vi "In_S2F23.vi"(8 "error in (no error)":errorcluster, 11 "S2 Message Class in":refnum<class "S2 Message Class.lvclass">) -> (0 "error out":errorcluster, 1 "OK?":bool, 2 "S2F23":T1, 3 "S2 Message Class out":refnum<class "S2 Message Class.lvclass">)   [LabVIEW 2020, in "SECS Communication.lvlib" / "S2 Message Class.lvclass"]
uses:
  S2 Message Class.lvclass
  D:/Dropbox/SECS/SECS_GEM v1.0.6/Com/SECS Communication/SECS-II Class/SECS-II Class.lvclass
  S2F23.ctl
  SECS-II Class/SECS-II Class.lvclass/SECS-II Class.ctl
  SECS-II Class/Variant To Data_U4.vi
  SECS-II Class/Variant To Data_ASCII.vi
  SECS-II Class/SECS-II Class.lvclass
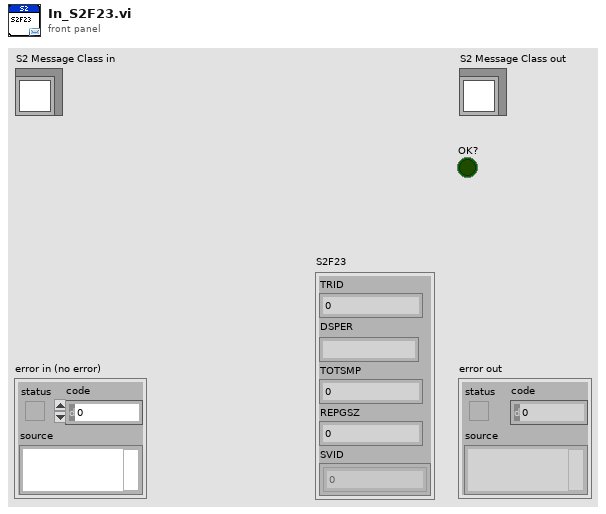
[diagram p1: front panel]
types:
  T1 = typedef "SECS Communication.lvlib/S2 Message Class.lvclass/S2F23.ctl" = cluster{"TRID":u32, "DSPER":string, "TOTSMP":u32, "REPGSZ":u32, "SVID":u32[]}
  T2 = typedef "SECS Communication.lvlib/SECS-II Class.lvclass/Message Data.ctl" = cluster{"Index":i32, "Data Item Format":T3, "Format Code":T4, "Parent Index":i32, "Child Index":i32[], "Data":variant}
  T3 = typedef "SECS Communication.lvlib/SECS-II Class.lvclass/Data Item Format.ctl" = enum16{"Data Type", "Value"}
  T4 = typedef "SECS Communication.lvlib/SECS-II Class.lvclass/Format Code.ctl" = enum16{"L", "A", "B", "Boolean", "J", "I1", "I2", "I4", "I8", "U1", "U2", "U4", "U8", "F4", "F8", "Char"}
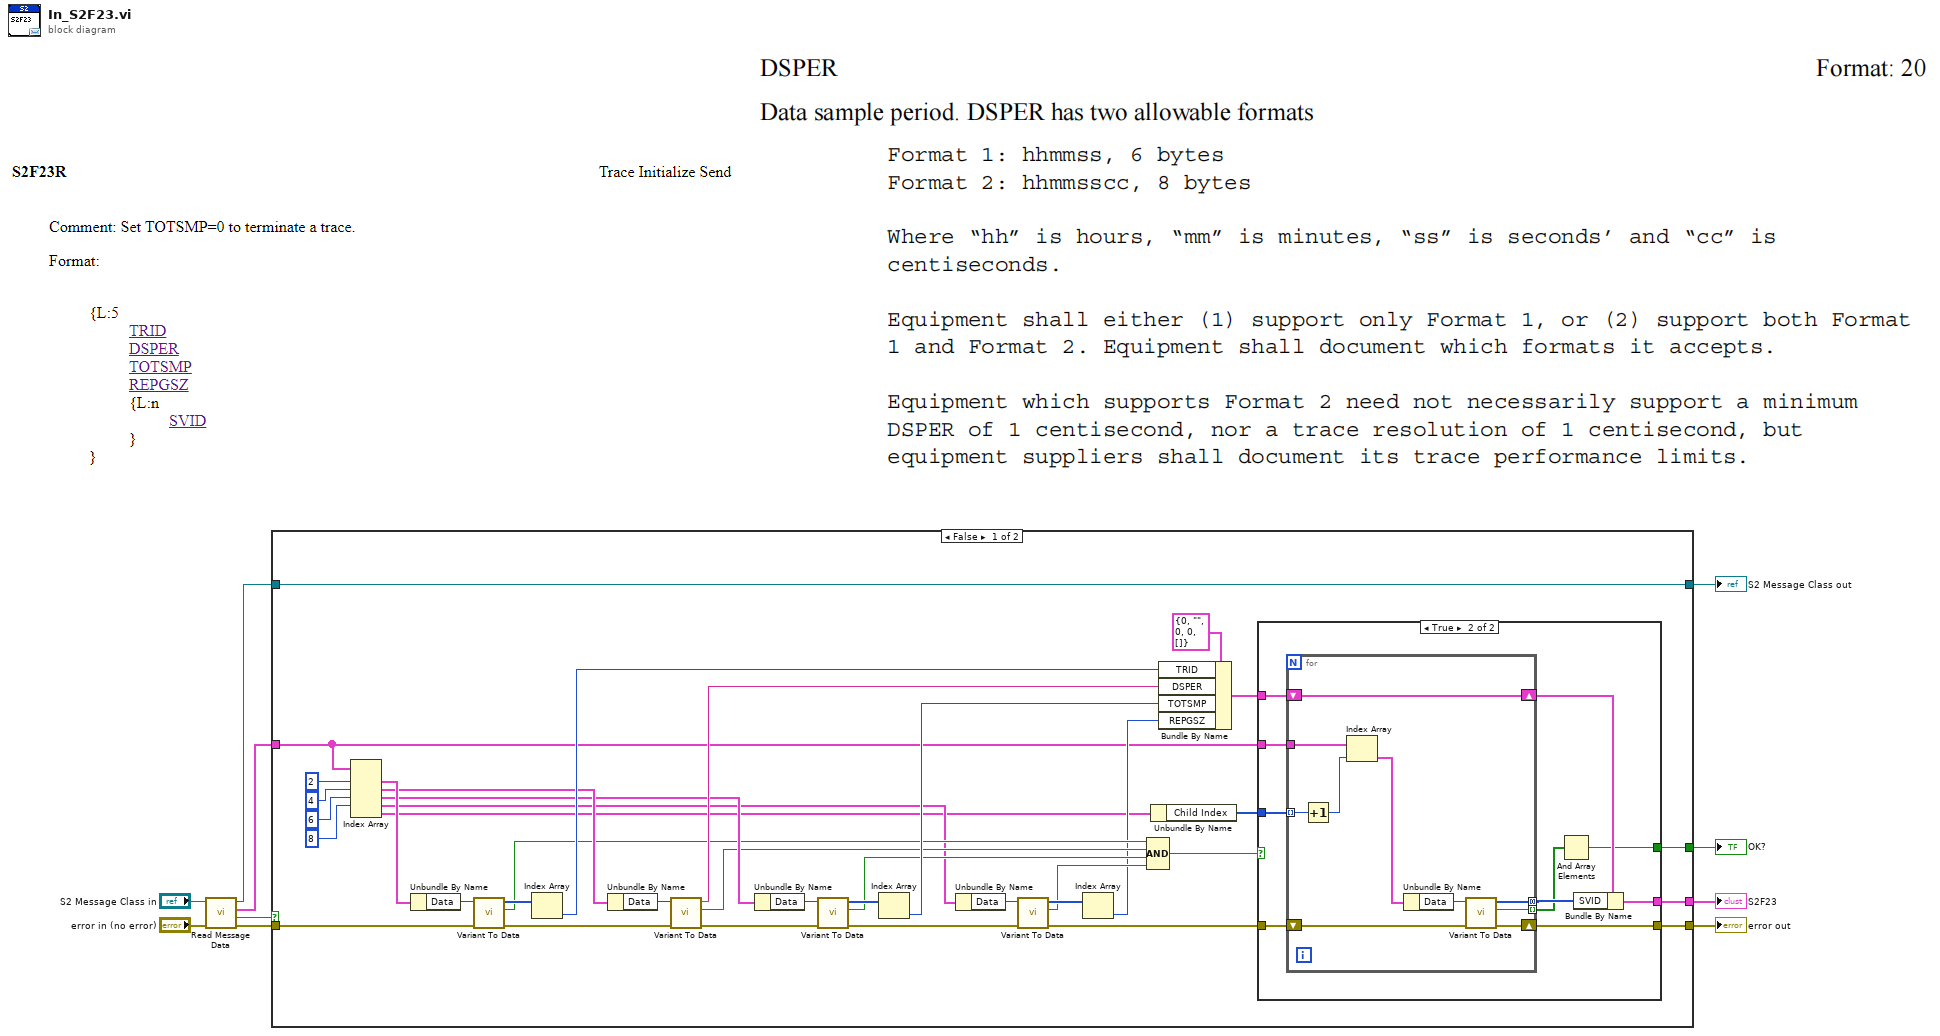
[diagram p0: block diagram]
diagram:
  n1 = call "Read Message Data.vi"("error in (no error)"="error in (no error)", "SECS-II Class in"="S2 Message Class in") -> ("error out"=w10:errorcluster, "Empty?"=w9:bool, "Message Data"=w8:T2[], "SECS-II Class out"=w7:refnum<class "S2 Message Class.lvclass">)  [unwired: 6 in]
  n2 = case shown="False" w9 {
    tunnel: w8 -> [w14 _]
    tunnel: w10 -> [w48 w70]
    tunnel: [w13 w70] -> w5
    tunnel: w7 -> [w47 w71]
    tunnel: [w47 w71] -> w1
    tunnel: [w12 _] -> w4
    tunnel: [w11 _] -> w6
    frame False {
      n3 = Index Array(array=w14, index #1=2 ("index"), index #2=4 ("index"), index #3=6 ("index"), index #4=8 ("index")) -> (element #1=w46:T2, element #2=w37:T2, element #3=w32:T2, element #4=w21:T2, element #5=w17:T2)  [unwired: 1 in]
      n4 = Unbundle By Name(w46) -> ("Data"=w45:variant)
      n5 = call-poly "Variant To Data.vi"("error in (no error)"=w48, "Variant"=w45) -> ("error out"=w38:errorcluster, "OK?"=w29:bool, "Data"=w42:u32[])  [unwired: 7 in]
      n6 = Index Array(array=w42) -> (element=w41:u32)  [unwired: 1 in]
      n7 = Unbundle By Name(w37) -> ("Data"=w39:variant)
      n8 = call-poly "Variant To Data.vi"("error in (no error)"=w38, "Variant"=w39) -> ("error out"=w34:errorcluster, "OK?"=w28:bool, "Data"=w36:string)  [unwired: 7 in]
      n9 = Unbundle By Name(w32) -> ("Data"=w35:variant)
      n10 = call-poly "Variant To Data.vi"("error in (no error)"=w34, "Variant"=w35) -> ("error out"=w23:errorcluster, "OK?"=w27:bool, "Data"=w30:u32[])  [unwired: 7 in]
      n11 = Index Array(array=w30) -> (element=w31:u32)  [unwired: 1 in]
      n12 = Unbundle By Name(w21) -> ("Data"=w24:variant)
      n13 = call-poly "Variant To Data.vi"("error in (no error)"=w23, "Variant"=w24) -> ("error out"=w19:errorcluster, "OK?"=w22:bool, "Data"=w25:u32[])  [unwired: 7 in]
      n14 = Index Array(array=w25) -> (element=w20:u32)  [unwired: 1 in]
      n15 = Compound Arithmetic op=AND(w29, w28, w27, w22) -> (w18:bool)
      n16 = Unbundle By Name(w17) -> ("Child Index"=w16:i32[])
      n17 = Bundle By Name(cluster=T1 {"TRID"=0, "DSPER"="", "TOTSMP"=0, "REPGSZ"=0, "SVID"=[]} ("S2F23"), "TRID"=w41, "DSPER"=w36, "TOTSMP"=w31, "REPGSZ"=w20) -> (w15:T1)
      n18 = case shown="True" w18 {
        tunnel: w19 -> [w49 w56]
        tunnel: w16 -> [_ w58]
        tunnel: w15 -> [_ w59]
        tunnel: w14 -> [_ w57]
        tunnel: [w49 w53] -> w13
        tunnel: [_ w51] -> w12
        tunnel: [_ w50] -> w11
        frame False {
        }
        frame True {
          n19 = for {
            shift-right: [w63] -> w55
            shift-left: w59 -> [w63]
            tunnel: w58 -> [w68] mode=indexing
            tunnel: w57 -> [w69]
            shift-right: [w60] -> w53
            shift-left: w56 -> [w65]
            tunnel: [w62] -> w54 mode=concatenating
            tunnel: [w61] -> w52 mode=indexing
            n20 = Increment(x=w68) -> (x+1=w67:i32)
            n21 = Index Array(array=w69, index=w67) -> (element=w64:T2)
            n22 = Unbundle By Name(w64) -> ("Data"=w66:variant)
            n23 = call-poly "Variant To Data.vi"("error in (no error)"=w65, "Variant"=w66) -> ("error out"=w60:errorcluster, "OK?"=w61:bool, "Data"=w62:u32[])  [unwired: 7 in]
          }
          n24 = And Array Elements(Boolean array=w52) -> (logical AND=w51:bool)
          n25 = Bundle By Name(cluster=w55, "SVID"=w54) -> (w50:T1)
        }
      }
    }
    frame True {
    }
  }
  "error out" <- w5
  "S2 Message Class out" <- w1
  "S2F23" <- w6
  "OK?" <- w4
